vi "Pockels Cal-Dialogue & retry save.vi"(10 "Pockels Cal table":string[][](array[string]), 11 "Pockels cal file path":path) -> (0 "error out":errorcluster)   [LabVIEW 2020]
uses:
  Typedefs/Read Write Enum.ctl
  <userlib>/My Palettes.lib/Files & paths/Spreadsheet/Write To Spreadsheet File (string)-Mod.vi
  Globals/gl_Calibration globals.vi
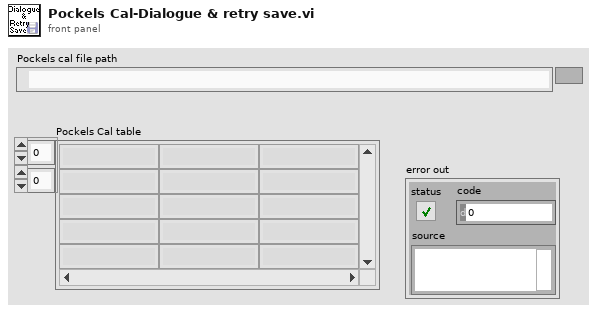
[diagram p1: front panel]
types:
  T1 = typedef "Read Write Enum.ctl" = enum16{"Read", "Write"}
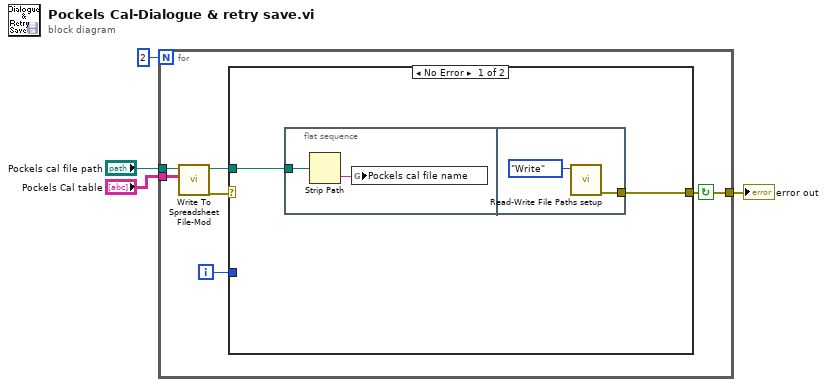
[diagram p0: block diagram]
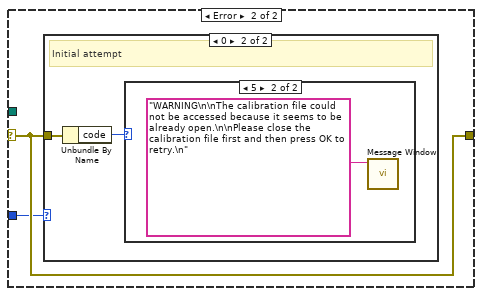
[diagram p2: hidden frame]
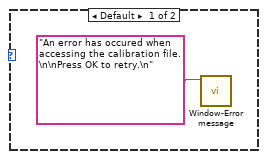
[diagram p4: hidden frame]
diagram:
  n1 = for {
    N: 2 -> [_]
    tunnel: [w6] -> w1
    tunnel: "Pockels Cal table" -> [w8]
    tunnel: "Pockels cal file path" -> [w7]
    i -> [w5]
    stop <- w6 continue-if-true
    n2 = call-poly <userlib>:"Write To Spreadsheet File-Mod.vi"("2D data"=w8, "file path (dialog if empty)"=w7) -> ("error out"=w10:errorcluster, "new file path (Not A Path if cancelled)"=w9:path)  [unwired: 8 in]
    n3 = case shown="No Error" w10 {
      selector: w10 -> [_ w18]
      tunnel: [w11 w18] -> w6
      tunnel: w9 -> [w12 _]
      tunnel: w5 -> [_ w17]
      frame No Error {
        n4 = flat-sequence {
          tunnel: w12 -> [w14]
          tunnel: [w15] -> w11
          frame #0 {
            n5 = Strip Path(path=w14) -> (name=w13:string)  [unwired: 1 out]
            n6 = global write "gl_Calibration globals.vi" "Pockels cal file name"(w13) -> ()
          }
          frame #1 {
            n7 = call "Read-Write File Paths setup.vi"("Function"=Read_Write_Enum."Write") -> ("error out"=w15:errorcluster)  [unwired: 10 in]
          }
        }
      }
      frame Error {
        n8 = case shown="0" w17 {
          tunnel: w18 -> [_ w20]
          frame Default {
            # "Consecutive attempt"
          }
          frame 0 {
            # "Initial attempt"
            n9 = Unbundle By Name(w20) -> ("code"=w19:i32)
            n10 = case shown="5" w19 {
              frame Default {
                n11 = call "Window-Error message.vi"("Message"="An error has occured when accessing the calibration file.\n\nPress OK to retry.\n") -> ()  [unwired: 10 in, 1 out]
              }
              frame 5 {
                n12 = call "Message Window.vi"("Message string"="WARNING\n\nThe calibration file could not be accessed because it seems to be already open.\n\nPlease close the calibration file first and then press OK to retry.\n" ("Message")) -> ()  [unwired: 10 in, 1 out]
              }
            }
          }
        }
      }
    }
  }
  "error out" <- w1
